vi "Send Command.vi"(6 "Command":T1, 8 "error in":errorcluster, 10 "Value":dbl, 11 "Luminos in":refnum<class "Luminos.lvclass">) -> (0 "error out":errorcluster, 3 "Luminos out":refnum<class "Luminos.lvclass">)   [LabVIEW 2018, in "Luminos.lvlib" / "Luminos.lvclass"]
uses:
  Luminos.lvclass
  PPLs/Axis/Axis.lvlibp/Custom Controls/Command.ctl
  PPLs/Axis/Axis.lvlibp/Axis.lvclass
  <instrlib>/ZaberTSeries/ZaberTSeries.lvlib
  C:/Projects/LabVIEW/PPLs/Axis/Axis.lvlibp/Axis.lvclass
  PPLs/Axis/Axis.lvlibp
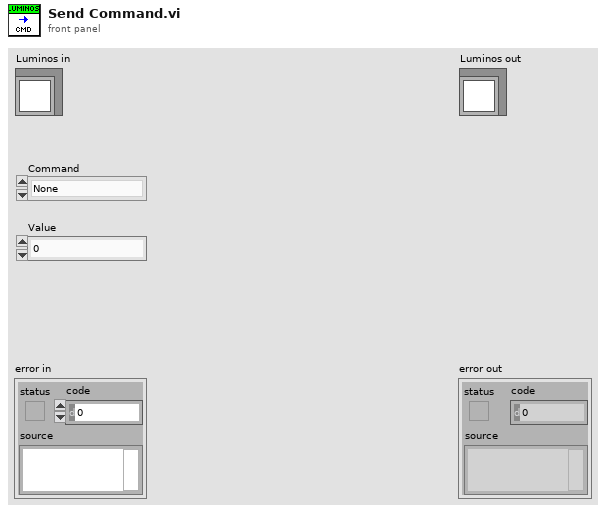
[diagram p1: front panel]
types:
  T1 = typedef "Axis.lvlibp/Command.ctl" = enum16{"None", "Home", "Renumber", "Move Absolute", "Move Relative", "Stop", "Set Run Speed", "Set Acceleration", "Set Run Current", "Set Home Offset", "Set Home Speed", "Query Current Position", "Load Defaults", "Query Status", "Lock Controls", "Unlock Controls"}
  T2 = typedef "ZaberTSeries.lvlib/Request.ctl" = cluster{"Device Number":u8, "Command":u8, "Data":i32, "Response Count":i32}
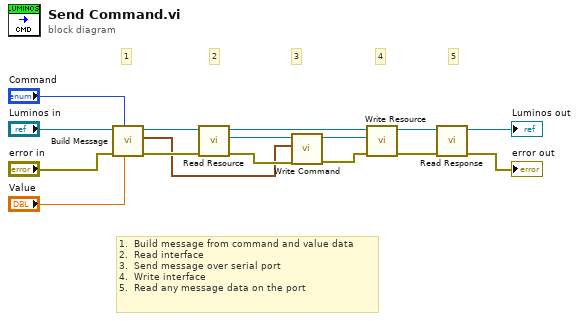
[diagram p0: block diagram]
diagram:
  # "1.  Build message from command and value data\n2.  Read interface\n3.  Send message over serial port\n4.  Write interface\n5.  Read any message data on the port"
  # "5"
  # "4"
  # "3"
  # "2"
  # "1"
  n1 = call "Build Message.vi"("Value"="Value", "Command"="Command", "error in"="error in", "Luminos in"="Luminos in") -> ("error out"=w9:errorcluster, "Message"=w7:T2, "Luminos out"=w11:refnum<class "Luminos.lvclass">)  [unwired: 5 in]
  n2 = call "Read Resource.vi"("error in"=w9, "Axis in"=w11) -> ("error out"=w13:errorcluster, "Resource"=w15:refnum<visa-resource-name>, "Axis out"=w16:refnum<class "Luminos.lvclass">)  [unwired: 7 in]
  n3 = call <instrlib>:"Write Command.vi"("error in (no error)"=w13, "Request"=w7, "VISA resource name"=w15) -> ("error out"=w12:errorcluster, "VISA resource name out"=w14:refnum<visa-resource-name>)  [unwired: 6 in, 1 out]
  n4 = call "Write Resource.vi"("error in"=w12, "Resource"=w14, "Axis in"=w16) -> ("error out"=w4:errorcluster, "Axis out"=w6:refnum<class "Luminos.lvclass">)  [unwired: 7 in]
  n5 = call-dynamic "Read Response.vi"("error in"=w4, "Luminos in"=w6) -> ("error out"=→"error out":errorcluster, "Luminos out"=→"Luminos out":refnum<class "Luminos.lvclass">)  [unwired: 7 in, 1 out]
